vi "Write.vi"(6 "Keep Bus Busy":bool, 7 "Timeout ms (1000)":i32=1000, 8 "error in (no error)":errorcluster, 9 "Bytes to Write":u8[](array[numeric]), 10 "Slave Address (7-bit)":u8, 11 "I2C Ref In":T1={"myRIO Reference"={"myRIO Model"=enum."Unknown", "myRIO Hardware Reference"={"Generic FPGA Reference"=refnum, "Allow multiple opens"=FALSE}}, "I2C Channels Enum"=enum."Not Connected", "I2C Configuration"={"I2C Transfer Rate"=enum."Fast mode (400 kbps)"}}) -> (0 "error out":errorcluster, 3 "I2C Ref Out":T1={"myRIO Reference"={"myRIO Model"=enum."Unknown", "myRIO Hardware Reference"={"Generic FPGA Reference"=refnum, "Allow multiple opens"=FALSE}}, "I2C Channels Enum"=enum."Not Connected", "I2C Configuration"={"I2C Transfer Rate"=enum."Fast mode (400 kbps)"}})   [LabVIEW 2021, in "I2C.lvlib"]
doc: "Writes data to an Inter-Integrated Circuit (I2C) slave device. This VI returns the result when finishing writing all the bytes or when timing out."
uses:
  <vilib>/myRIO/Instrument Drivers/Onboard IO/I2C/I2C.lvlib
  <vilib>/myRIO/Instrument Drivers/Onboard IO/I2C/typedefs/I2C Reference.ctl
  <vilib>/myRIO/Common/Instrument Driver Framework/Utilities/typedefs/myRIO Generic Hardware Reference.ctl
  <vilib>/myRIO/Common/Instrument Driver Framework/Utilities/typedefs/Hardware Version Enum.ctl
  <vilib>/myRIO/Common/Instrument Driver Framework/Utilities/typedefs/myRIO v1.0 Reference.ctl
  <vilib>/myRIO/Common/Instrument Driver Framework/Utilities/typedefs/Generic FPGA Reference.ctl
  <vilib>/myRIO/Common/Instrument Driver Framework/myRIO v1.0/I2C/typedefs/I2C Channels Enum.ctl
  <vilib>/myRIO/Instrument Drivers/Onboard IO/I2C/typedefs/I2C Configuration.ctl
  <vilib>/myRIO/Instrument Drivers/Onboard IO/I2C/typedefs/I2C Transfer Rate.ctl
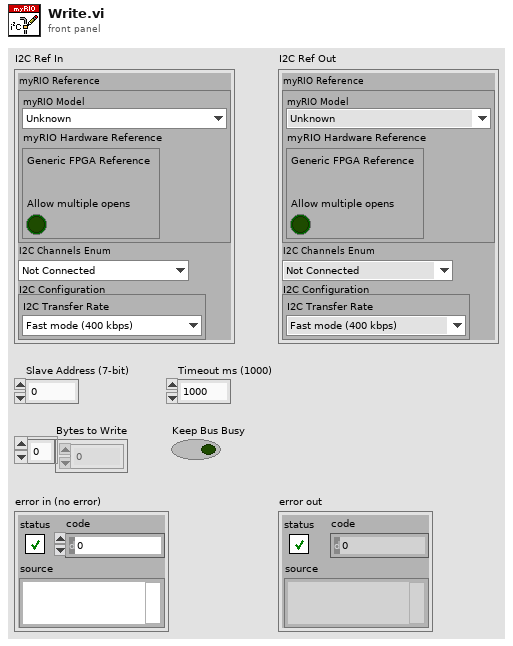
[diagram p1: front panel]
types:
  T1 = typedef "I2C.lvlib/I2C Reference.ctl" = cluster{"myRIO Reference":T2, "I2C Channels Enum":T6, "I2C Configuration":T7}
  T2 = typedef "myRIO Generic Hardware Reference.ctl" = cluster{"myRIO Model":T3, "myRIO Hardware Reference":T4}
  T3 = typedef "Hardware Version Enum.ctl" = enum16{"Unknown", "myRIO-1900", "myRIO-1950", "roboRIO", "NI ELVIS RIO CM", "ELVIS III"}
  T4 = typedef "myRIO v1.0 Reference.ctl" = cluster{"Generic FPGA Reference":T5, "Allow multiple opens":bool}
  T5 = typedef "Generic FPGA Reference.ctl" = refnum<k20>
  T6 = typedef "I2C Channels Enum.ctl" = enum16{"Not Connected", "A/I2C", "B/I2C", "I2C/I2C"}
  T7 = typedef "I2C.lvlib/I2C Configuration.ctl" = cluster{"I2C Transfer Rate":T8}
  T8 = typedef "I2C.lvlib/I2C Transfer Rate.ctl" = enum16{"Standard mode (100 kbps)", "Fast mode (400 kbps)"}
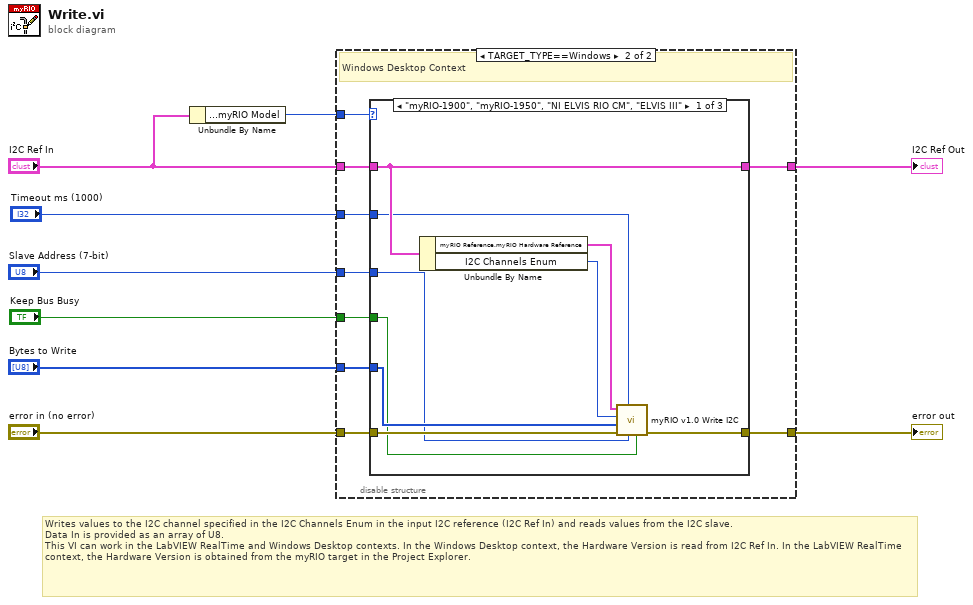
[diagram p0: block diagram]
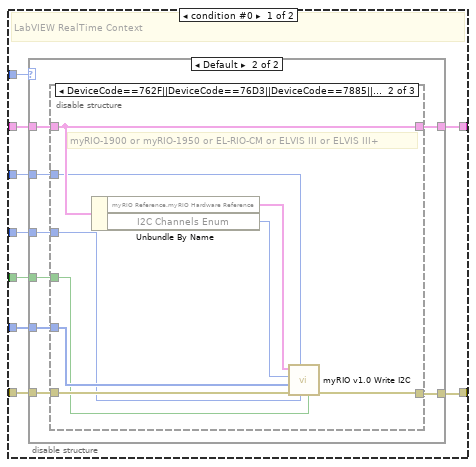
[diagram p2: hidden frame]
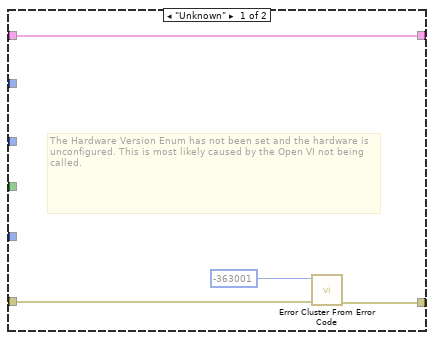
[diagram p3: hidden frame]
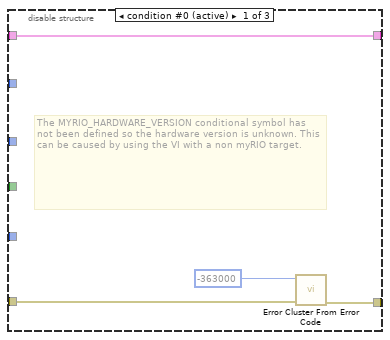
[diagram p4: hidden frame]
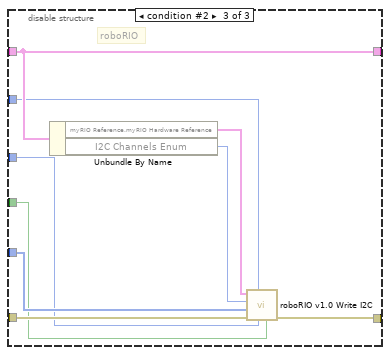
[diagram p5: hidden frame]
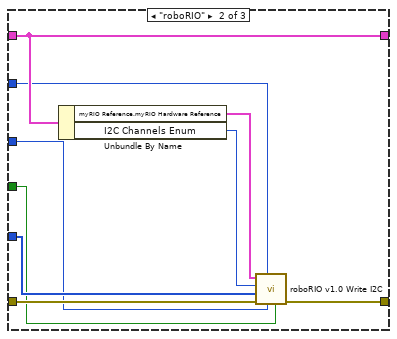
[diagram p6: hidden frame]
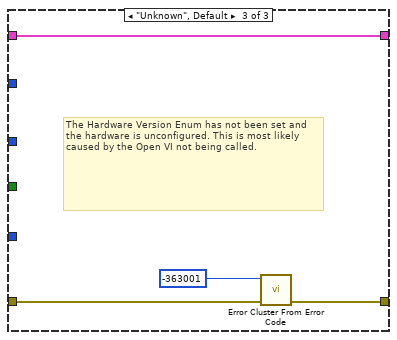
[diagram p7: hidden frame]
diagram:
  # "Writes values to the I2C channel specified in the I2C Channels Enum in the input I2C reference (I2C Ref In) and reads values from the I2C slave.\nData In is provided as an array of U8.\nThis VI can work in the LabVIEW RealTime and Windows Desktop contexts. In the Windows Desktop context, the Hardware Version is read from I2C Ref In. In the LabVIEW RealTime context, the Hardware Version is obtained from the myRIO target in the Project Explorer."
  n1 = Unbundle By Name("I2C Ref In") -> ("myRIO Reference.myRIO Model"=w3:T3)
  n2 = disable-structure shown="TARGET_TYPE==Windows" {
    disable-tunnel: [w18 w61] -> w6
    disable-tunnel: "I2C Ref In" -> [w17 w58]
    disable-tunnel: "error in (no error)" -> [w16 w60]
    disable-tunnel: [w15 w59] -> w7
    disable-tunnel: w3 -> [w14 w57]
    disable-tunnel: "Bytes to Write" -> [w13 w56]
    disable-tunnel: "Slave Address (7-bit)" -> [w12 w55]
    disable-tunnel: "Keep Bus Busy" -> [w11 w54]
    disable-tunnel: "Timeout ms (1000)" -> [w10 w53]
    frame condition #0 {
      # "LabVIEW RealTime Context"
      n3 = case shown="Default" w14 {
        tunnel: [w21 w30] -> w18
        tunnel: w17 -> [w19 w29]
        tunnel: w16 -> [w20 w28]
        tunnel: [w19 w27] -> w15
        tunnel: w13 -> [_ w26]
        tunnel: w12 -> [_ w25]
        tunnel: w11 -> [_ w24]
        tunnel: w10 -> [_ w23]
        frame "Unknown" {
          # "The Hardware Version Enum has not been set and the hardware is unconfigured. This is most likely caused by the Open VI not being called."
          n4 = call <vilib>:"Error Cluster From Error Code.vi"("error in (no error)"=w20, "error code (0)"=-363001) -> ("error out"=w21:errorcluster)  [unwired: 7 in]
        }
        frame Default {
          n5 = disable-structure shown="DeviceCode==762F||DeviceCode==76D3||DeviceCode==7885||DeviceCode==7928||DeviceCode==793C" {
            disable-tunnel: w29 -> [w31 w41 w50]
            disable-tunnel: [w34 w39 w48] -> w30
            disable-tunnel: w28 -> [w32 w40 w49]
            disable-tunnel: [w31 w41 w50] -> w27
            disable-tunnel: w26 -> [_ w38 w47]
            disable-tunnel: w25 -> [_ w37 w46]
            disable-tunnel: w24 -> [_ w36 w45]
            disable-tunnel: w23 -> [_ w35 w44]
            frame condition #0 (active) {
              # "The MYRIO_HARDWARE_VERSION conditional symbol has not been defined so the hardware version is unknown. This can be caused by using the VI with a non myRIO target."
              n6 = call <vilib>:"Error Cluster From Error Code.vi"("error in (no error)"=w32, "error code (0)"=-363000) -> ("error out"=w34:errorcluster)  [unwired: 7 in]
            }
            frame condition #1 {
              # "myRIO-1900 or myRIO-1950 or EL-RIO-CM or ELVIS III or ELVIS III+"
              n7 = Unbundle By Name(w41) -> ("myRIO Reference.myRIO Hardware Reference"=w43:T4, "I2C Channels Enum"=w42:T6)
              n8 = call <vilib>:"myRIO v1.0 Write I2C.vi"("Keep Bus Busy"=w36, "Slave Address (7-bit)"=w37, "Timeout ms (1000)"=w35, "Error In (No Error)"=w40, "Data to Write"=w38, "Channel"=w42, "myRIO Ref In"=w43) -> ("error out"=w39:errorcluster)  [unwired: 3 in, 1 out]
            }
            frame condition #2 {
              # "roboRIO"
              n9 = Unbundle By Name(w50) -> ("myRIO Reference.myRIO Hardware Reference"=w52:T4, "I2C Channels Enum"=w51:T6)
              n10 = call <vilib>:"roboRIO v1.0 Write I2C.vi"("Keep Bus Busy"=w45, "Slave Address (7-bit)"=w46, "Timeout ms (1000)"=w44, "Error In (No Error)"=w49, "Data to Write"=w47, "Channel"=w51, "myRIO Ref In"=w52) -> ("error out"=w48:errorcluster)  [unwired: 3 in, 1 out]
            }
          }
        }
      }
    }
    frame condition #1 (active) {
      # "Windows Desktop Context"
      n11 = case shown="\"myRIO-1900\", \"myRIO-1950\", \"NI ELVIS RIO CM\", \"ELVIS III\"" w57 {
        tunnel: [w67 w76 w83] -> w61
        tunnel: w58 -> [w68 w77 w80]
        tunnel: w60 -> [w66 w75 w81]
        tunnel: [w68 w77 w80] -> w59
        tunnel: w56 -> [w65 w74 _]
        tunnel: w55 -> [w64 w73 _]
        tunnel: w54 -> [w63 w72 _]
        tunnel: w53 -> [w62 w71 _]
        frame "myRIO-1900", "myRIO-1950", "NI ELVIS RIO CM", "ELVIS III" {
          n12 = Unbundle By Name(w68) -> ("myRIO Reference.myRIO Hardware Reference"=w70:T4, "I2C Channels Enum"=w69:T6)
          n13 = call <vilib>:"myRIO v1.0 Write I2C.vi"("Keep Bus Busy"=w63, "Slave Address (7-bit)"=w64, "Timeout ms (1000)"=w62, "Error In (No Error)"=w66, "Data to Write"=w65, "Channel"=w69, "myRIO Ref In"=w70) -> ("error out"=w67:errorcluster)  [unwired: 3 in, 1 out]
        }
        frame "roboRIO" {
          n14 = Unbundle By Name(w77) -> ("myRIO Reference.myRIO Hardware Reference"=w79:T4, "I2C Channels Enum"=w78:T6)
          n15 = call <vilib>:"roboRIO v1.0 Write I2C.vi"("Keep Bus Busy"=w72, "Slave Address (7-bit)"=w73, "Timeout ms (1000)"=w71, "Error In (No Error)"=w75, "Data to Write"=w74, "Channel"=w78, "myRIO Ref In"=w79) -> ("error out"=w76:errorcluster)  [unwired: 3 in, 1 out]
        }
        frame "Unknown", Default {
          # "The Hardware Version Enum has not been set and the hardware is unconfigured. This is most likely caused by the Open VI not being called."
          n16 = call <vilib>:"Error Cluster From Error Code.vi"("error in (no error)"=w81, "error code (0)"=-363001) -> ("error out"=w83:errorcluster)  [unwired: 7 in]
        }
      }
    }
  }
  "I2C Ref Out" <- w7
  "error out" <- w6
